vi "config handler.vi"(7 "Operation":enum16{"Open", "Write", "Read", "Close"}(ring), 8 "error in (no error)":errorcluster, 10 "Write values":T1, 11 "Part number (.ini)":string) -> (0 "Error Out":errorcluster, 2 "Read values":T1)   [LabVIEW 2021]
uses:
  <vilib>/Utility/config.llb/Write Key (String).vi
  <vilib>/Utility/config.llb/Read Key (String).vi
  <vilib>/Utility/config.llb/NI_LVConfig.lvlib
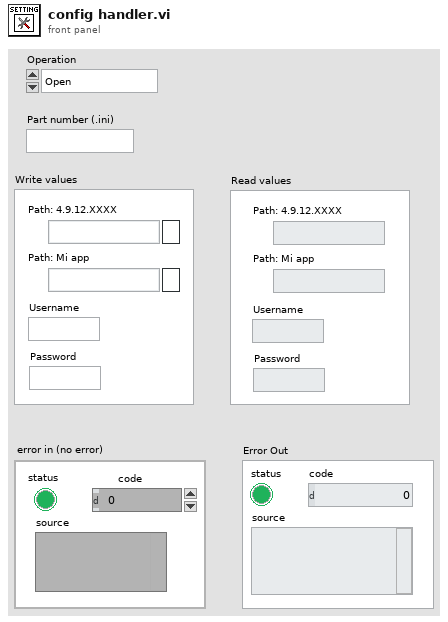
[diagram p1: front panel]
types:
  T1 = cluster{"Path: 4.9.12.XXXX":path, "Path: Mi app":path, "Username":string, "Password":string}
  T2 = typedef "NI_LVConfig.lvlib/Config Data RefNum.ctl" = refnum<k1>
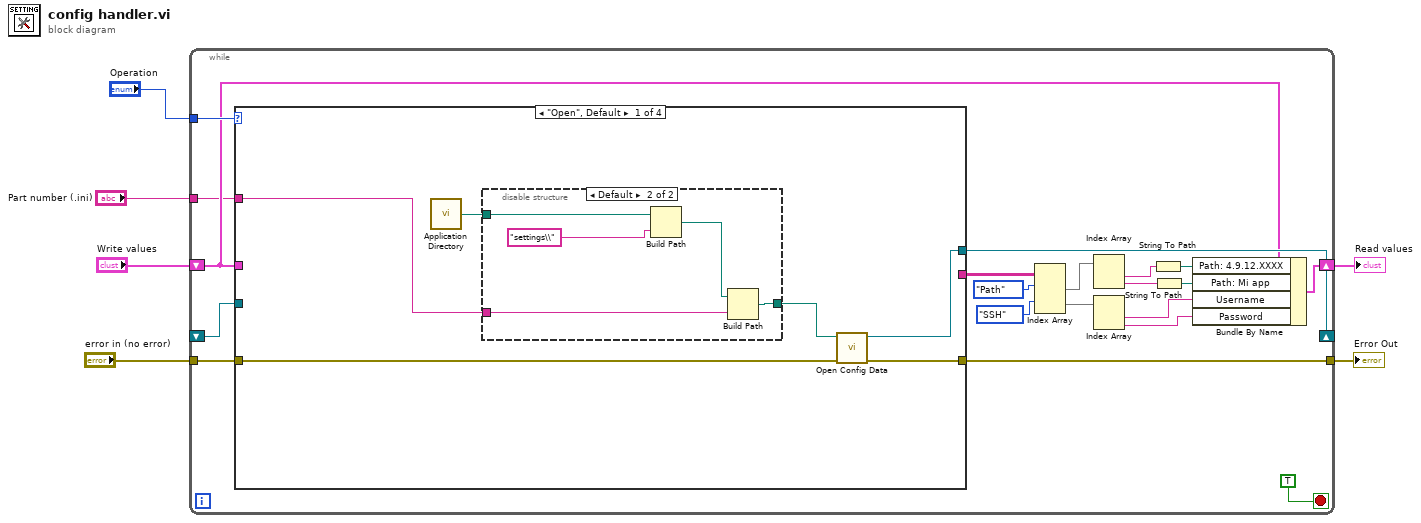
[diagram p0: block diagram]
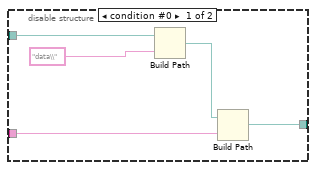
[diagram p2: hidden frame]
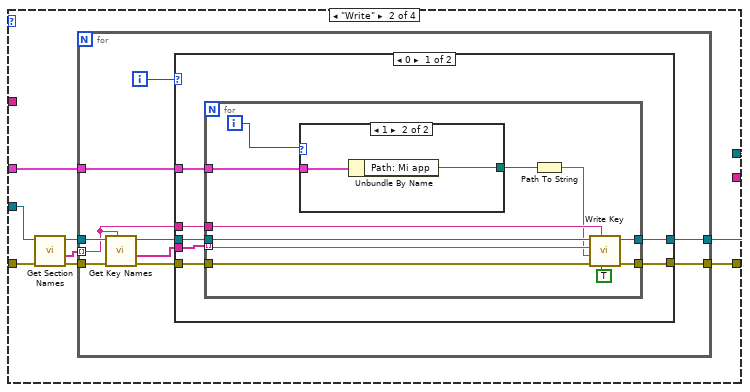
[diagram p3: hidden frame]
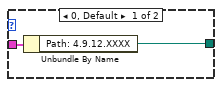
[diagram p4: hidden frame]
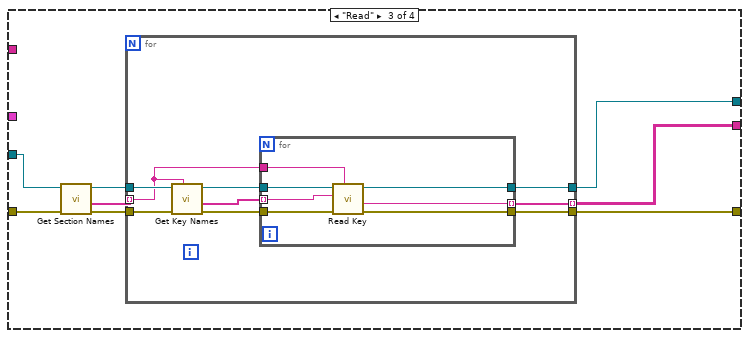
[diagram p6: hidden frame]
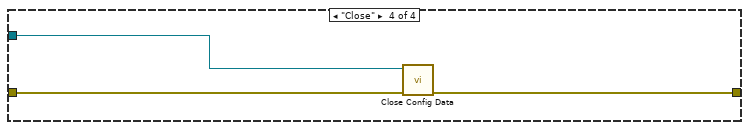
[diagram p7: hidden frame]
diagram:
  n1 = while {
    tunnel: "error in (no error)" -> [w26]
    tunnel: [w25] -> w5
    shift-right: [w24] -> _
    shift-left: _ -> [w22]
    tunnel: "Operation" -> [w21]
    shift-right: [w17] -> w2
    shift-left: "Write values" -> [w20]
    tunnel: "Part number (.ini)" -> [w7]
    stop <- TRUE stop-if-true
    n2 = case shown="\"Open\", Default" w21 {
      tunnel: w26 -> [w32 w47 w91 w111]
      tunnel: [w31 w44 w86 w110] -> w25
      tunnel: [w30 w45 w87 _] -> w24
      tunnel: w22 -> [_ w46 w92 w109]
      tunnel: w20 -> [_ w43 _ _]
      tunnel: [_ _ w85 _] -> w16
      tunnel: w7 -> [w27 _ _ _]
      frame "Open", Default {
        n3 = call <vilib>:"Application Directory.vi"() -> ("Application Directory"=w29:path)
        n4 = disable-structure shown="Default" {
          disable-tunnel: [w33 w40] -> w28
          disable-tunnel: w29 -> [w36 w41]
          disable-tunnel: w27 -> [w34 w38]
          frame condition #0 {
            n5 = Build Path(base path=w36, name or relative path="data\\") -> (appended path=w35:path)
            n6 = Build Path(base path=w35, name or relative path=w34) -> (appended path=w33:path)
          }
          frame condition #1 (active) {
            n7 = Build Path(base path=w41, name or relative path="settings\\") -> (appended path=w39:path)
            n8 = Build Path(base path=w39, name or relative path=w38) -> (appended path=w40:path)
          }
        }
        n9 = call <vilib>:"Open Config Data.vi"("error in (no error)"=w32, "configuration file path"=w28) -> ("error out"=w31:errorcluster, "refnum"=w30:T2)  [unwired: 7 in, 1 out]
      }
      frame "Write" {
        n10 = call <vilib>:"Get Section Names.vi"("error in (no error)"=w47, "refnum"=w46) -> ("error out"=w48:errorcluster, "section names"=w50:string[], "refnum out"=w49:T2)  [unwired: 7 in]
        n11 = for {
          tunnel: w50 -> [w58] mode=indexing
          tunnel: w49 -> [w60]
          tunnel: w48 -> [w59]
          tunnel: [w54] -> w45
          tunnel: [w53] -> w44
          tunnel: w43 -> [w52]
          i -> [w51]
          n12 = call <vilib>:"Get Key Names.vi"("section"=w58, "error in (no error)"=w59, "refnum"=w60) -> ("error out"=w55:errorcluster, "key names"=w57:string[], "refnum out"=w56:T2)  [unwired: 5 in, 1 out]
          n13 = case shown="0" w51 {
            tunnel: w58 -> [w67 _]
            tunnel: w57 -> [w66 _]
            tunnel: w56 -> [w65 w83]
            tunnel: w55 -> [w64 w84]
            tunnel: [w63 w83] -> w54
            tunnel: [w62 w84] -> w53
            tunnel: w52 -> [w61 _]
            frame 0 {
              n14 = for {
                tunnel: w67 -> [w78]
                tunnel: w66 -> [w77] mode=indexing
                tunnel: w65 -> [w76]
                tunnel: w64 -> [w75]
                tunnel: [w74] -> w63
                tunnel: [w73] -> w62
                tunnel: w61 -> [w72]
                i -> [w68]
                n15 = case shown="1" w68 {
                  tunnel: w72 -> [w80 w82]
                  tunnel: [w79 w81] -> w69
                  frame 0, Default {
                    n16 = Unbundle By Name(w80) -> ("Path: 4.9.12.XXXX"=w79:path)
                  }
                  frame 1 {
                    n17 = Unbundle By Name(w82) -> ("Path: Mi app"=w81:path)
                  }
                }
                n18 = Path To String(path=w69) -> (string=w71:string)
                n19 = call-poly <vilib>:"Write Key.vi"("write raw string? (F)"=TRUE, "section"=w78, "error in (no error)"=w75, "value"=w71, "key"=w77, "refnum"=w76) -> ("error out"=w73:errorcluster, "refnum out"=w74:T2)  [unwired: 3 in, 1 out]
              }
            }
            frame 2, Default {
            }
          }
        }
      }
      frame "Read" {
        n20 = call <vilib>:"Get Section Names.vi"("error in (no error)"=w91, "refnum"=w92) -> ("error out"=w88:errorcluster, "section names"=w90:string[], "refnum out"=w89:T2)  [unwired: 7 in]
        n21 = for {
          tunnel: w90 -> [w99] mode=indexing
          tunnel: w89 -> [w101]
          tunnel: w88 -> [w100]
          tunnel: [w95] -> w87
          tunnel: [w94] -> w86
          tunnel: [w93] -> w85 mode=indexing
          n22 = call <vilib>:"Get Key Names.vi"("section"=w99, "error in (no error)"=w100, "refnum"=w101) -> ("error out"=w96:errorcluster, "key names"=w98:string[], "refnum out"=w97:T2)  [unwired: 5 in, 1 out]
          n23 = for {
            tunnel: w99 -> [w108]
            tunnel: w98 -> [w107] mode=indexing
            tunnel: w97 -> [w106]
            tunnel: w96 -> [w105]
            tunnel: [w104] -> w95
            tunnel: [w103] -> w94
            tunnel: [w102] -> w93 mode=indexing
            n24 = call-poly <vilib>:"Read Key.vi"("section"=w108, "error in (no error)"=w105, "key"=w107, "refnum"=w106) -> ("error out"=w103:errorcluster, "value"=w102:string, "refnum out"=w104:T2)  [unwired: 4 in, 1 out]
          }
        }
      }
      frame "Close" {
        n25 = call <vilib>:"Close Config Data.vi"("error in (no error)"=w111, "refnum"=w109) -> ("error out"=w110:errorcluster)  [unwired: 8 in, 1 out]
      }
    }
    n26 = Index Array(array=w16, index (row) #1=enum16{"Path", "SSH", "Idle"}."Path", index (row) #2=enum16{"Path", "SSH", "Idle"}."SSH") -> (element #1=w13:string[], element #2=w11:string[])  [unwired: 2 in]
    n27 = Index Array(array=w13) -> (element #1=w12:string, element #2=w9:string)  [unwired: 2 in]
    n28 = Index Array(array=w11) -> (element #1=w10:string, element #2=w8:string)  [unwired: 2 in]
    n29 = String To Path(string=w12) -> (path=w18:path)
    n30 = String To Path(string=w9) -> (path=w19:path)
    n31 = Bundle By Name(cluster=w20, "Path: 4.9.12.XXXX"=w18, "Path: Mi app"=w19, "Username"=w10, "Password"=w8) -> (w17:T1)
  }
  "Error Out" <- w5
  "Read values" <- w2
